vi "Dialog Window with Option.vi"(8 "Error In":errorcluster, 9 "Button 2 (Cancel)":string="Cancel", 10 "Button 1 (OK)":string="OK", 11 "Message":string) -> (0 "Error Out":errorcluster, 1 "Cancelled?":bool, 3 "OK?":bool)   [LabVIEW 2021, in "GUI.lvlib"]
uses:
  GUI.lvlib
panel:
  in  "Cancel":bool
  in  "OK":bool
  in  "Do not show this warning again":bool
  out "Displayed Message":string
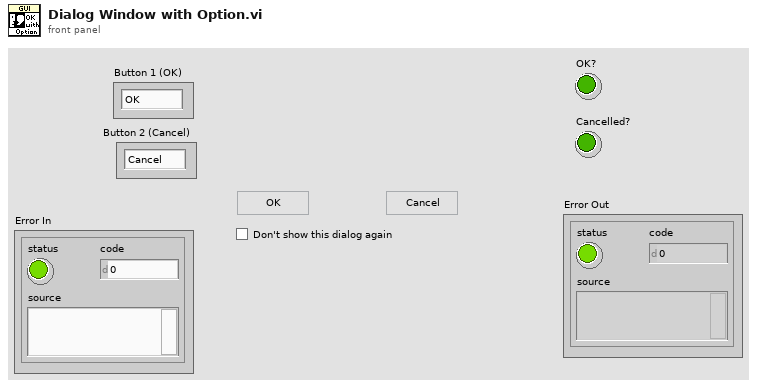
[diagram p1: front panel]
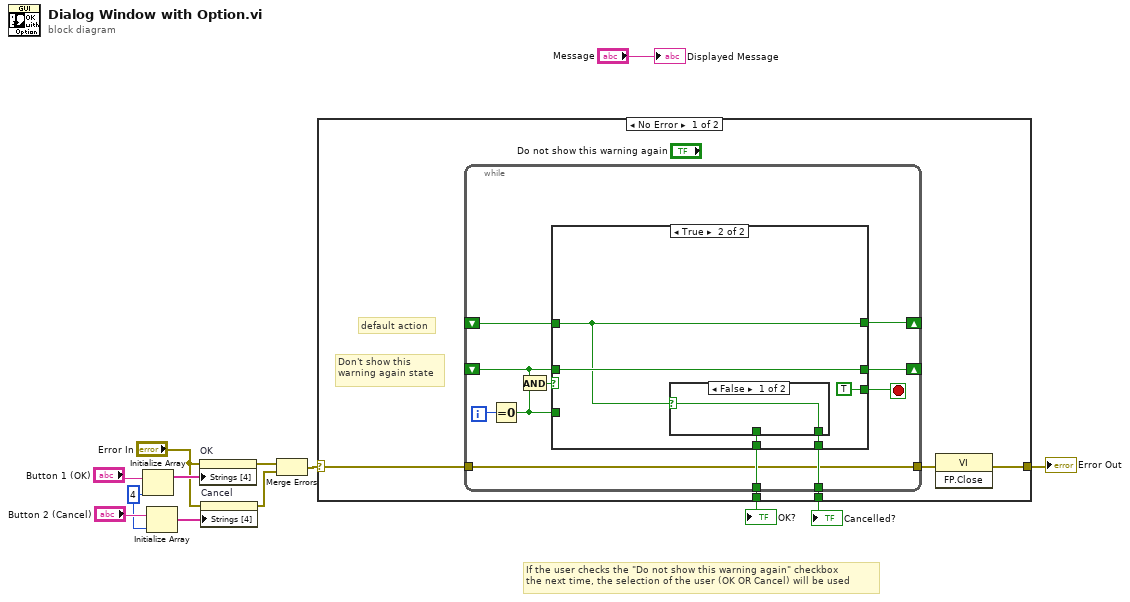
[diagram p0: block diagram]
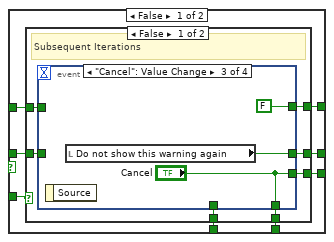
[diagram p2: hidden frame]
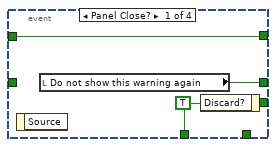
[diagram p3: hidden frame]
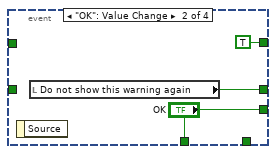
[diagram p4: hidden frame]
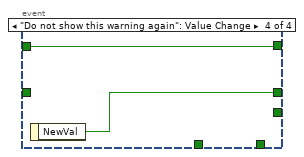
[diagram p5: hidden frame]
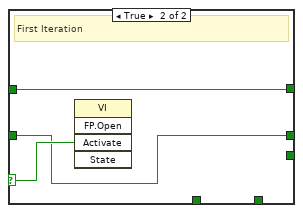
[diagram p6: hidden frame]
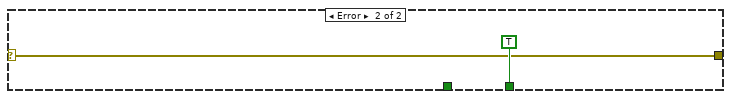
[diagram p8: hidden frame]
diagram:
  w7 = 4 ("dimension size")
  # "If the user checks the \"Do not show this warning again\" checkbox\nthe next time, the selection of the user (OK OR Cancel) will be used"
  n1 = Initialize Array("Button 1 (OK)", w7) -> (w9:string[])
  n2 = Initialize Array("Button 2 (Cancel)", w7) -> (w6:string[])
  n3 = property on="OK" class="Bool"(error in="Error In", "Strings [4]"=w9) -> (error out=w2:errorcluster)  [unwired: 1 in, 1 out]
  n4 = property on="Cancel" class="Bool"(error in="Error In", "Strings [4]"=w6) -> (error out=w1:errorcluster)  [unwired: 1 in, 1 out]
  n5 = Merge Errors(w2, w1) -> (w3:errorcluster)
  n6 = case shown="No Error" w3 {
    selector: w3 -> [w16 w66]
    tunnel: [w18 _] -> w12
    tunnel: [w17 TRUE ("Cancel")] -> w11
    tunnel: [w14 w66] -> w5
    frame No Error {
      # "Don't show this warning again state"
      # "default action"
      n7 = while {
        shift-right: [w29] -> _
        shift-left: _ -> [w27]
        tunnel: [w23] -> w18
        tunnel: [w22] -> w17
        shift-right: [w21] -> _
        shift-left: _ -> [w20]
        tunnel: w16 -> [w19]
        tunnel: [w19] -> w15
        i -> [w28]
        stop <- w25 stop-if-true
        n8 = Equal To 0?(x=w28) -> (x = 0?=w24:bool)
        n9 = And(x=w27, y=w24) -> (x .and. y?=w26:bool)
        n10 = case shown="False" w26 {
          tunnel: [w37 TRUE ("Cancel")] -> w25
          tunnel: [w36 w62] -> w29
          tunnel: w27 -> [w35 w62]
          tunnel: w24 -> [w34 _]
          tunnel: [w33 w60] -> w23
          tunnel: [w32 w59] -> w22
          tunnel: [w31 w61] -> w21
          tunnel: w20 -> [w30 w61]
          frame False {
            n11 = case shown="False" w34 {
              selector: w34 -> [_ w58]
              tunnel: [w44 _] -> w37
              tunnel: [w43 w57] -> w36
              tunnel: w35 -> [w42 w57]
              tunnel: [w41 _] -> w33
              tunnel: [w40 _] -> w32
              tunnel: [w39 w56] -> w31
              tunnel: w30 -> [w38 w56]
              frame False {
                # "Subsequent Iterations"
                n12 = event shown="[2] \"Cancel\": Value Change" {
                  selector: _ -> [_ _ _ _]
                  dyn-events: _ -> [_ _ _ _]
                  timeout: _ -> [_ _ _ _]
                  tunnel: [w46 "OK" "Cancel" _] -> w44
                  tunnel: [w47 w50 w52 w55] -> w43
                  tunnel: w42 -> [_ _ _ _]
                  tunnel: [w46 "OK" _ _] -> w41
                  tunnel: [_ _ "Cancel" _] -> w40
                  tunnel: [w45 TRUE ("Cancel") FALSE ("Cancel") w54] -> w39
                  tunnel: w38 -> [w45 _ _ w54]
                  event Panel Close? {
                    w46 = TRUE ("Discard?")
                    n13 = event-data() -> ()  [unwired: 1 in, 1 out]
                    n14 = local read "Do not show this warning again"() -> (w47:bool)
                    n15 = event-data("Discard?"=w46) -> ()  [unwired: 1 in, 1 out]
                  }
                  event "OK": Value Change {
                    n16 = event-data() -> ()  [unwired: 1 in, 1 out]
                    n17 = local read "Do not show this warning again"() -> (w50:bool)
                  }
                  event "Cancel": Value Change {
                    n18 = event-data() -> ()  [unwired: 1 in, 1 out]
                    n19 = local read "Do not show this warning again"() -> (w52:bool)
                  }
                  event "Do not show this warning again": Value Change {
                    n20 = event-data() -> ("NewVal"=w55:bool)  [unwired: 1 in]
                  }
                }
              }
              frame True {
                # "First Iteration"
                n21 = invoke class="VI" method="FP.Open"("Activate"=w58) -> ()  [unwired: 4 in, 5 out]
              }
            }
          }
          frame True {
            n22 = case shown="False" w61 {
              selector: w61 -> [w64 w65]
              tunnel: [_ w65] -> w60
              tunnel: [w64 _] -> w59
              frame False {
              }
              frame True {
              }
            }
          }
        }
      }
      n23 = invoke class="VI" method="FP.Close"(error in=w15) -> (error out=w14:errorcluster)  [unwired: 2 in, 2 out]
    }
    frame Error {
    }
  }
  "OK?" <- w12
  "Cancelled?" <- w11
  "Error Out" <- w5
  "Displayed Message" <- "Message"
